vi "main.vi"() -> ()   [LabVIEW 2026, in "G-AI Core.lvlib"]
uses:
  G-AI Core.lvlib
  <vilib>/jgoebel/LabVIEW MCP Server SDK/MCP Server.lvlib
panel:
  out "Log":string
  # "Keep this VI open to make the G-AI MCP-Server reachable from your\nMCP Client (e.g. Claude Desktop).\nAdd MCP Server to mcp_config.json or claude_desktop_config.json"
  # "Server Name: G-AI\nServer Port: 36987\nServer URL: /mcp/server"
  # "https://github.com/JanGoebel/G-AI"
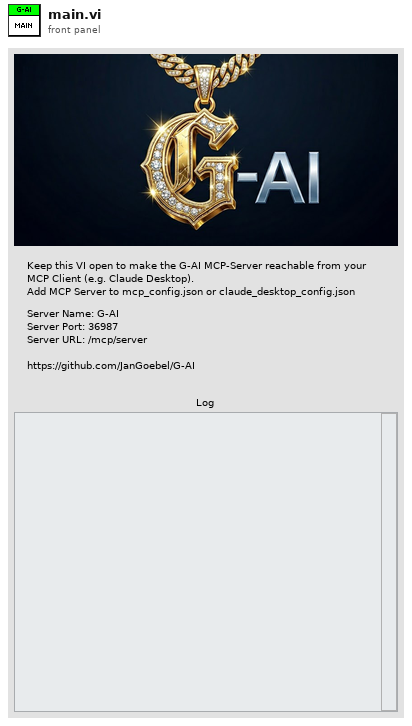
[diagram p1: front panel]
types:
  T1 = typedef "MCP Server.lvlib/User Events.ctl" = cluster{"onError":refnum<user-event>, "onRpc":refnum<user-event>}
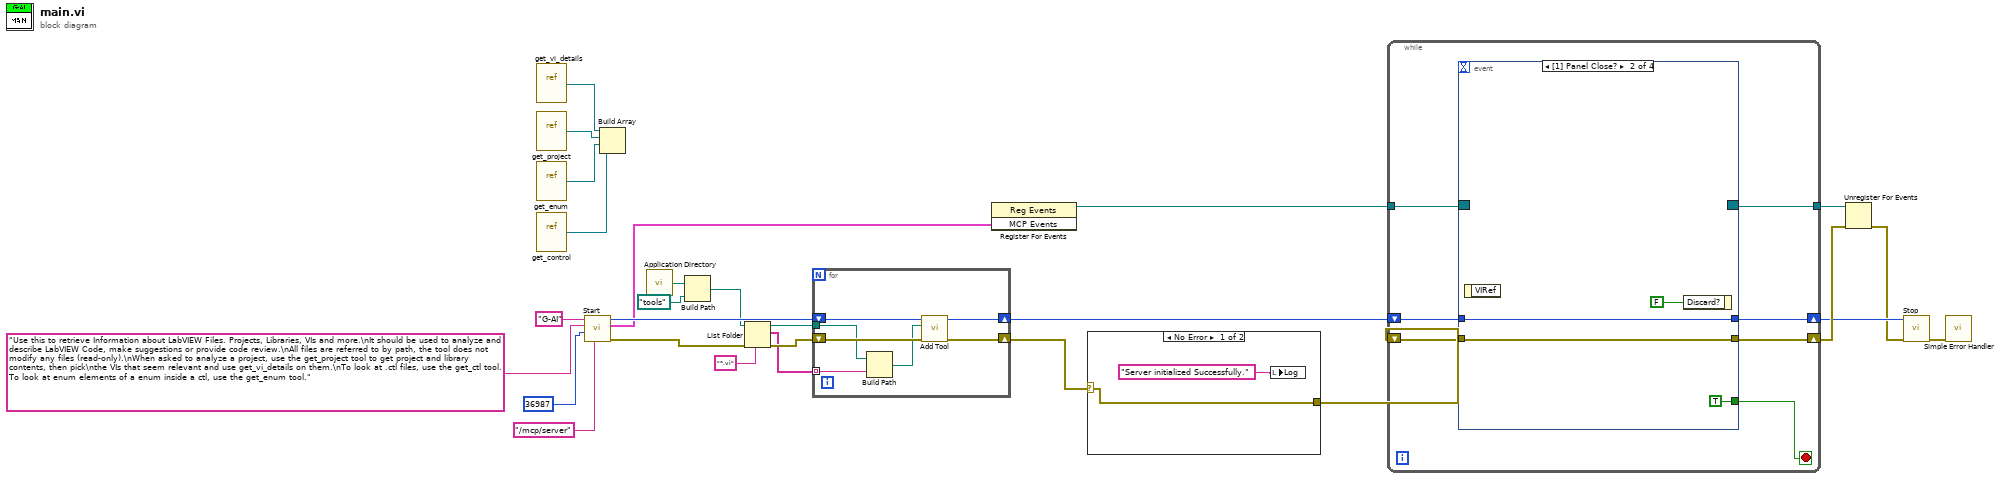
[diagram p0: block diagram]
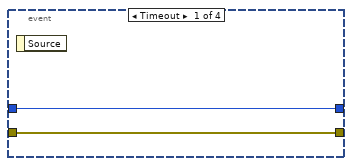
[diagram p3: hidden frame]
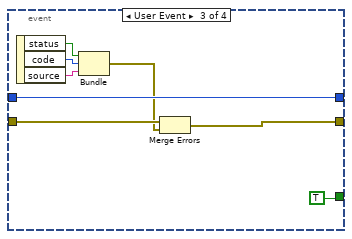
[diagram p4: hidden frame]
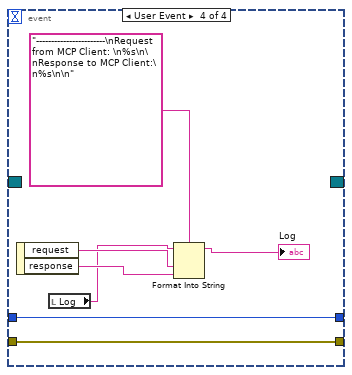
[diagram p5: hidden frame]
diagram:
  n1 = vi-ref "get_vi_details.vi"() -> (w21:refnum<vi>)
  n2 = vi-ref "get_project.vi"() -> (w20:refnum<vi>)
  n3 = vi-ref "get_enum.vi"() -> (w19:refnum<vi>)
  n4 = vi-ref "get_control.vi"() -> (w8:refnum<vi>)
  n5 = call <vilib>:"Start.vi"("url (\"/mcp/server\")"="/mcp/server" ("url (\"/mcp/server\")"), "HTTP Port (36987)"=u16 36987, "Description"="Use this to retrieve Information about LabVIEW Files. Projects, Libraries, VIs and more.\nIt should be used to analyze and describe LabVIEW Code, make suggestions or provide code review.\nAll files are referred to by path, the tool does not modify any files (read-only).\nWhen asked to analyze a project, use the get_project tool to get project and library contents, then pick\nthe VIs that seem relevant and use get_vi_details on them.\nTo look at .ctl files, use the get_ctl tool. To look at enum elements of a enum inside a ctl, use the get_enum tool.", "Name"="G-AI") -> ("error out"=w26:errorcluster, "MCP Events"=w16:T1, "server id out"=w27:i32)  [unwired: 5 in]
  n6 = Build Array(w21, w20, w19, w8) -> ()  [unwired: 1 out]
  n7 = call <vilib>:"Application Directory.vi"() -> ("Application Directory"=w7:path)
  n8 = Build Path(base path=w7, name or relative path=path "tools") -> (appended path=w4:path)
  n9 = List Folder(path=w4, pattern="*.vi", error in=w26) -> (path out=w2:path, filenames=w1:string[], error out=w5:errorcluster)  [unwired: 1 in, 1 out]
  n10 = for {
    shift-right: [w32] -> w25
    shift-left: w27 -> [w34]
    shift-right: [w31] -> w9
    shift-left: w5 -> [w33]
    tunnel: w2 -> [w29]
    tunnel: w1 -> [w30] mode=indexing
    n11 = Build Path(base path=w29, name or relative path=w30) -> (appended path=w28:path)
    n12 = call <vilib>:"Add Tool.vi"("error in (no error)"=w33, "vi path"=w28, "server id"=w34) -> ("error out"=w31:errorcluster, "server id out"=w32:i32)  [unwired: 7 in]
  }
  n13 = register-events(w16) -> (reference out=w15:refnum<event-registration>)  [unwired: 2 in, 1 out]
  n14 = case shown="No Error" w9 {
    selector: w9 -> [w35 w37]
    tunnel: [w35 w37] -> w10
    frame No Error {
      n15 = local write "Log"("Server initialized Successfully." ("Log")) -> ()
    }
    frame Error {
    }
  }
  n16 = while {
    shift-right: [w41] -> w17
    shift-left: w25 -> [w44]
    shift-right: [w42] -> w18
    shift-left: w10 -> [w43]
    tunnel: w15 -> [w40]
    tunnel: [w38] -> w13
    stop <- w39 stop-if-true
    n17 = event shown="[1] Panel Close?" {
      selector: w40 -> [_ _ _ _]
      dyn-events: [_ _ _ _] -> w38
      timeout: _ -> [_ _ _ _]
      tunnel: w44 -> [w46 w48 w57 w64]
      tunnel: w43 -> [w45 w47 w58 w65]
      tunnel: [w45 w47 w52 w65] -> w42
      tunnel: [w46 w48 w57 w64] -> w41
      tunnel: [_ TRUE TRUE _] -> w39
      event Timeout {
        n18 = event-data() -> ()  [unwired: 1 in, 1 out]
      }
      event Panel Close? {
        n19 = event-data() -> ()  [unwired: 1 in, 1 out]
        n20 = event-data("Discard?"=FALSE) -> ()  [unwired: 1 in, 1 out]
      }
      event User Event {
        n21 = event-data() -> ("status"=w55:bool, "code"=w54:i32, "source"=w53:string)  [unwired: 1 in]
        n22 = Bundle("status"=w55, "code"=w54, "source"=w53) -> (w51:errorcluster)  [unwired: 1 in]
        n23 = Merge Errors(w58, w51) -> (w52:errorcluster)
      }
      event User Event {
        n24 = event-data() -> ("request"=w62:string, "response"=w61:string)  [unwired: 1 in]
        n25 = local read "Log"() -> (w60:string)
        n26 = Format Into String(format string="-----------------------\nRequest from MCP Client: \n%s\n\nResponse to MCP Client:\n%s\n\n", initial string=w60, w62, w61) -> (resulting string=→"Log":string)  [unwired: 1 in, 1 out]
      }
    }
  }
  n27 = Unregister For Events(event registration refnum=w13, error in=w18) -> (error out=w14:errorcluster)
  n28 = call <vilib>:"Stop.vi"("error in (no error)"=w14, "id"=w17) -> ("error out"=w12:errorcluster)  [unwired: 9 in]
  n29 = call <vilib>:"Simple Error Handler.vi"("error in (no error)"=w12) -> ()  [unwired: 4 in, 5 out]
